vi "Configure Trigger (NFC - Trigger Event).vi"(7 "Arm Event (0: None)":i32(ring) items=["None", "ASR", "AALL", "AEIT", "BSR", "BALL", "BEIT", "FSR"], 8 "error in (no error)":errorcluster, 9 "Standard (0: A)":i32(ring) items=["A", "A106", "B", "B106", "F212", "F424"], 10 "Trigger Event (3: AEIT)":i32(ring)=3 items=["ATR", "ASR", "AALL", "AEIT", "ASDD", "BSR", "BALL", "BEIT", "ATT", "FSR", "FAR", "FPR"], 11 "VISA resource name":refnum<visa-resource-name>) -> (0 "error out":errorcluster, 3 "VISA resource name out":refnum<visa-resource-name>)   [LabVIEW 2017, in "Agilent 2000 3000 X-Series.lvlib"]
doc: "Configures the trigger event for NFC (Near Field Communication). \n\n<b>Note:</b>\nThis VI is only applicable for 3000T, 3000G, 4000 X-Series."
uses:
  Agilent 2000 3000 X-Series.lvlib
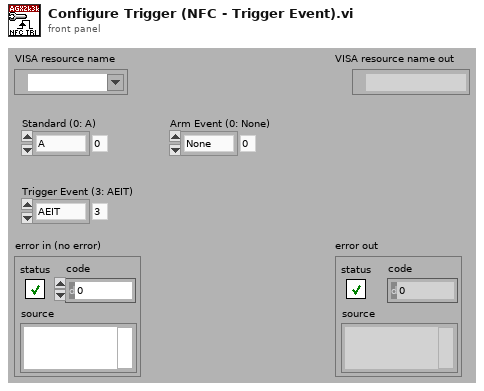
[diagram p1: front panel]
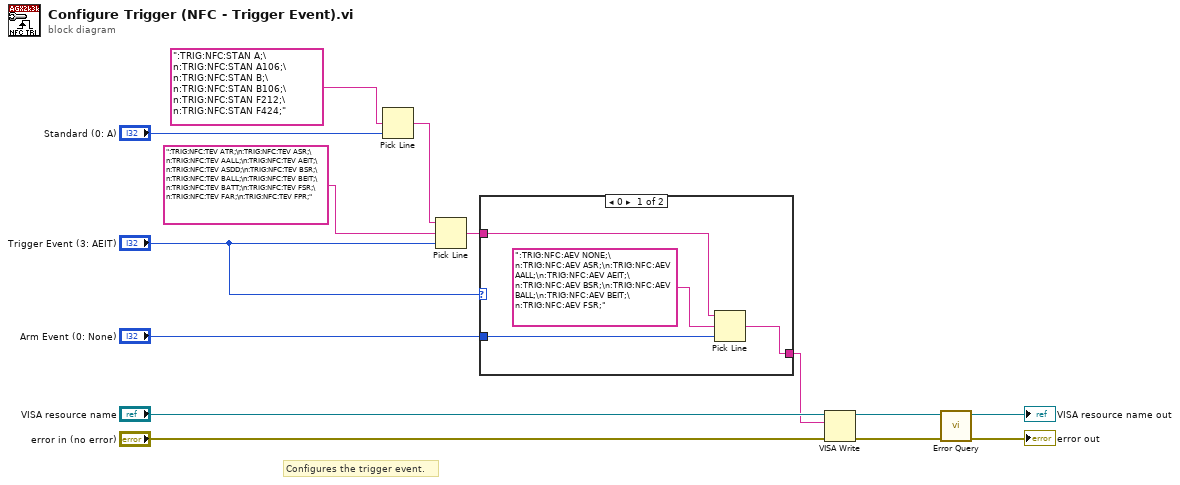
[diagram p0: block diagram]
diagram:
  # "Configures the trigger event."
  n1 = Pick Line(multi-line string=":TRIG:NFC:STAN A;\n:TRIG:NFC:STAN A106;\n:TRIG:NFC:STAN B;\n:TRIG:NFC:STAN B106;\n:TRIG:NFC:STAN F212;\n:TRIG:NFC:STAN F424;", line index="Standard (0: A)") -> (output string=w6:string)  [unwired: 1 in]
  n2 = Pick Line(string ("")=w6, multi-line string=":TRIG:NFC:TEV ATR;\n:TRIG:NFC:TEV ASR;\n:TRIG:NFC:TEV AALL;\n:TRIG:NFC:TEV AEIT;\n:TRIG:NFC:TEV ASDD;\n:TRIG:NFC:TEV BSR;\n:TRIG:NFC:TEV BALL;\n:TRIG:NFC:TEV BEIT;\n:TRIG:NFC:TEV BATT;\n:TRIG:NFC:TEV FSR;\n:TRIG:NFC:TEV FAR;\n:TRIG:NFC:TEV FPR;", line index="Trigger Event (3: AEIT)") -> (output string=w7:string)
  n3 = case shown="0" "Trigger Event (3: AEIT)" {
    tunnel: "Arm Event (0: None)" -> [w17 _]
    tunnel: w7 -> [w16 w19]
    tunnel: [w15 w19] -> w1
    frame 0 {
      n4 = Pick Line(string ("")=w16, multi-line string=":TRIG:NFC:AEV NONE;\n:TRIG:NFC:AEV ASR;\n:TRIG:NFC:AEV AALL;\n:TRIG:NFC:AEV AEIT;\n:TRIG:NFC:AEV BSR;\n:TRIG:NFC:AEV BALL;\n:TRIG:NFC:AEV BEIT;\n:TRIG:NFC:AEV FSR;", line index=w17) -> (output string=w15:string)
    }
    frame 1..11, Default {
    }
  }
  n5 = VISA Write(VISA resource name="VISA resource name", write buffer=w1, error in (no error)="error in (no error)") -> (VISA resource name out=w5:refnum<visa-resource-name>, error out=w4:errorcluster)  [unwired: 1 out]
  n6 = call "Error Query.vi"("error in (no error)"=w4, "VISA resource name"=w5) -> ("error out"=→"error out":errorcluster, "VISA resource name out"=→"VISA resource name out":refnum<visa-resource-name>)  [unwired: 6 in, 2 out]
